vi "判断整除2.vi"(1 "被除数":dbl, 2 "除数":dbl) -> (0 "布尔 2":bool)   [LabVIEW 2013]
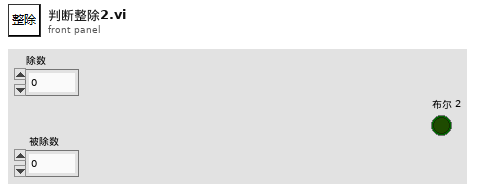
[diagram p1: front panel]
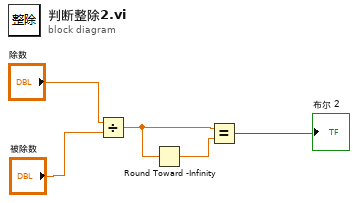
[diagram p0: block diagram]
diagram:
  n1 = Divide(x="除数", y="被除数") -> (x/y=w3:dbl)
  n2 = Round Toward -Infinity(1:w3) -> (0:w2:dbl)
  n3 = Equal?(x=w3, y=w2) -> (x = y?=→"布尔 2":bool)
